vi "Daqmx_List.vi"(0 "Device Number n":u8) -> (1 "NI-DAQmx Device Names":tag[](array[tag]), 2 "NI-DAQmx Device Types":string[](array[string]), 3 "Number of NI-DAQmx Devices":i32, 4 "NI-DAQmx Device Name n":tag)   [LabVIEW 2019]
uses:
  <resource>/objmgr/daqmx.rc
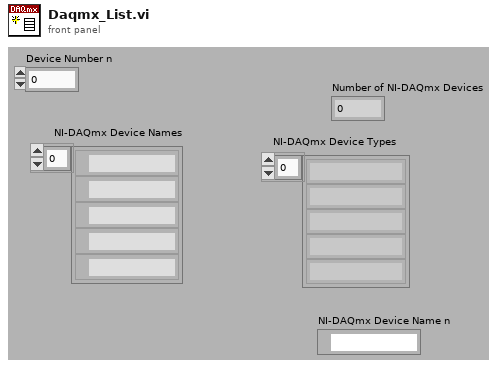
[diagram p1: front panel]
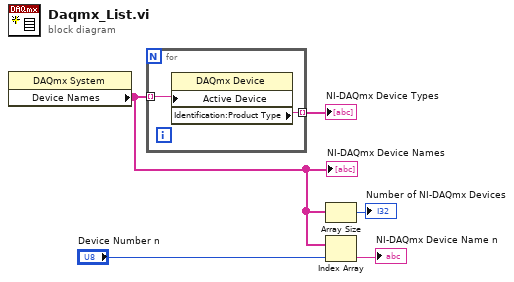
[diagram p0: block diagram]
diagram:
  n1 = property class="DAQmx System"() -> ("Device Names"=w3:tag[])  [unwired: 2 in, 2 out]
  "NI-DAQmx Device Names" <- w3
  n2 = for {
    tunnel: w3 -> [w7] mode=indexing
    tunnel: [w6] -> w5 mode=indexing
    n3 = property class="DAQmx Device"("Active Device"=w7) -> ("Identification:Product Type"=w6:string)  [unwired: 2 in, 2 out]
  }
  "NI-DAQmx Device Types" <- w5
  n4 = Array Size(array=w3) -> (size(s)=→"Number of NI-DAQmx Devices":i32)
  n5 = Index Array(array=w3, index="Device Number n") -> (element=→"NI-DAQmx Device Name n":tag)
